vi "Panel Resized.vi"(6 "Sizing Refnums":T2, 8 "error in (no error)":errorcluster, 9 "Origin":cluster{"H":i16, "V":i16}, 10 "NewBnds":T1, 11 "Size Constraints":cluster{"min tab width":i32, "w/h":dbl}) -> (0 "error out":errorcluster)   [LabVIEW 2023]
uses:
  <vilib>/Utility/miscctls.llb/LVRectTypeDef.ctl
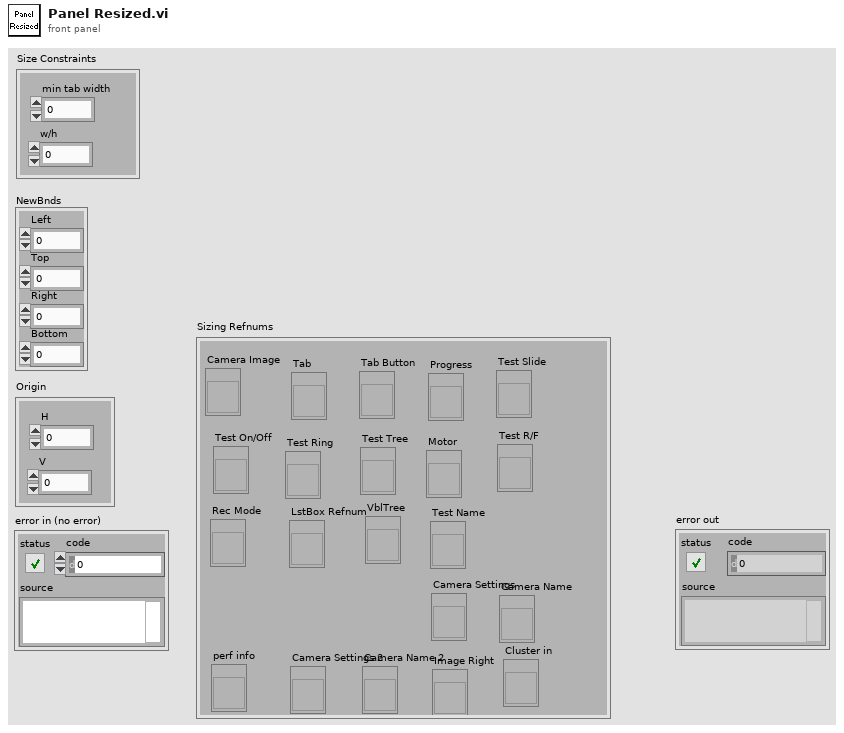
[diagram p1: front panel]
types:
  T1 = typedef "LVRectTypeDef.ctl" = cluster{"Left":i16, "Top":i16, "Right":i16, "Bottom":i16}
  T2 = cluster{"Camera Image":refnum<vi>, "Tab":refnum<vi>, "Tab Button":refnum<vi>, "Rec Mode":refnum<vi>, "Test Slide":refnum<vi>, "Test On/Off":refnum<vi>, "Test Ring":refnum<vi>, "Test R/F":refnum<vi>, "Test Name":refnum<vi>, "Motor":refnum<vi>, "Progress":refnum<vi>, "LstBox Refnum":refnum<vi>, "Test Tree":refnum<vi>, "VblTree":refnum<vi>, "Camera Settings":refnum<vi>, "Camera Name":refnum<vi>, "perf info":refnum<vi>, "Camera Settings 2":refnum<vi>, "Camera Name 2":refnum<vi>, "Image Right":refnum<vi>, "Cluster in":refnum<vi>}
  T3 = typedef "LVPositionTypeDef.ctl" = cluster{"Left":i32, "Top":i32}
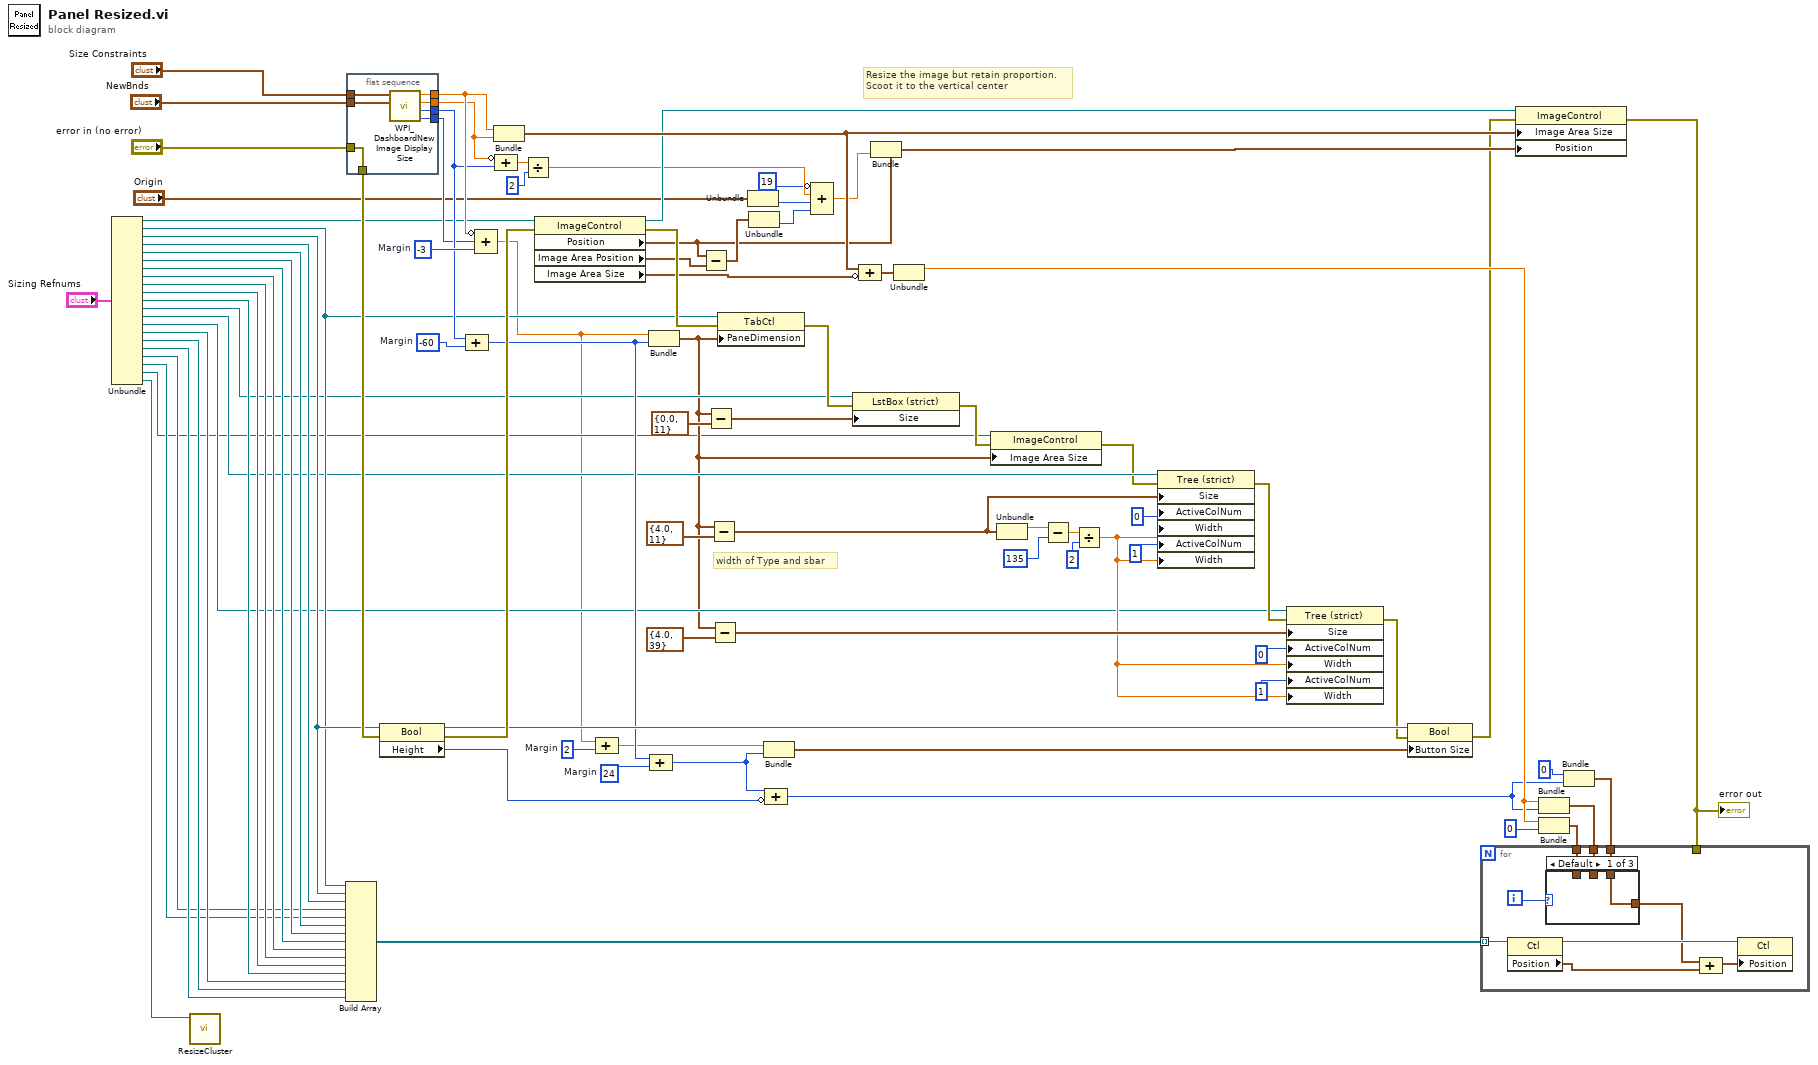
[diagram p0: block diagram]
diagram:
  w77 = 24  # Margin
  w75 = 2  # Margin
  w72 = -60  # Margin
  w81 = -3  # Margin
  # "width of Type and sbar"
  # "Resize the image but retain proportion.\nScoot it to the vertical center"
  n1 = Unbundle("Sizing Refnums") -> ("Camera Image"=w46:refnum<vi>, "Tab"=w47:refnum<vi>, "Tab Button"=w55:refnum<vi>, "Rec Mode"=w23:refnum<vi>, "Test Slide"=w22:refnum<vi>, "Test On/Off"=w21:refnum<vi>, "Test Ring"=w20:refnum<vi>, "Test R/F"=w19:refnum<vi>, "Test Name"=w18:refnum<vi>, "Motor"=w17:refnum<vi>, "Progress"=w16:refnum<vi>, "LstBox Refnum"=w15:refnum<vi>, "Test Tree"=w14:refnum<vi>, "VblTree"=w13:refnum<vi>, "Camera Settings"=w10:refnum<vi>, "Camera Name"=w9:refnum<vi>, "perf info"=w8:refnum<vi>, "Camera Settings 2"=w7:refnum<vi>, "Camera Name 2"=w6:refnum<vi>, "Image Right"=w3:refnum<vi>, "Cluster in"=w1:refnum<vi>)
  n2 = call "ResizeCluster.vi"("Cluster in"=w1) -> ()  [unwired: 11 in]
  n3 = Build Array(w47, w55, w23, w7, w6, w22, w21, w20, w19, w18, w17, w16, w10, w9, w8) -> (w90:refnum<vi>[])
  n4 = flat-sequence {
    tunnel: "NewBnds" -> [w97]
    tunnel: "Size Constraints" -> [w96]
    tunnel: [w95] -> w71
    tunnel: [w94] -> w78
    tunnel: [w93] -> w79
    tunnel: [w92] -> w80
    tunnel: [w91] -> w89
    tunnel: "error in (no error)" -> [w91]
    frame #0 {
      n5 = call <vilib>:"WPI_DashboardNew Image Display Size.vi"("NewBnds"=w97, "Size Constraints"=w96) -> ("Window Width"=w95:i16, "Window Height"=w93:i16, "Height"=w94:dbl, "Width"=w92:dbl)  [unwired: 6 in]
    }
  }
  n6 = property class="Bool"(reference=w55, error in=w89) -> (reference out=w84:refnum<vi>, error out=w88:errorcluster, "Height"=w83:u32)
  n7 = Compound Arithmetic op=unknown(w79, w72) -> (w76:i32)
  n8 = Compound Arithmetic op=ADD(invert w80, w71, w81) -> (w2:dbl)
  n9 = Bundle("Width"=w80, "Height"=w78) -> (w67:cluster{"Width":dbl, "Height":dbl})  [unwired: 1 in]
  n10 = Compound Arithmetic op=ADD(invert w78, w79) -> (w59:dbl)
  n11 = Divide(x=w59, y=2) -> (x/y=w61:dbl)
  n12 = property class="ImageControl"(reference=w46, error in=w88) -> (reference out=w64:refnum<vi>, error out=w87:errorcluster, "Position"=w63:T3, "Image Area Position"=w58:cluster{"Left":i32, "Top":i32}, "Image Area Size"=w69:cluster{"Width":u32, "Height":u32})
  n13 = Compound Arithmetic op=ADD(w2, w75) -> (w74:dbl)
  n14 = Bundle(w2, w76) -> (w12:cluster{dbl, i32})  [unwired: 1 in]
  n15 = Compound Arithmetic op=ADD(w76, w77) -> (w82:i32)
  n16 = Subtract(x=w63, y=w58) -> (x-y=w65:T3)
  n17 = Subtract(x=w12, y=cluster{dbl, i32} {0.0, 11}) -> (x-y=w44:cluster{dbl, i32})
  n18 = Subtract(x=w12, y=cluster{dbl, i32} {4.0, 11}) -> (x-y=w35:cluster{dbl, i32})
  n19 = Subtract(x=w12, y=cluster{dbl, i32} {4.0, 39}) -> (x-y=w40:cluster{dbl, i32})
  n20 = property class="TabCtl"(reference=w47, error in=w87, "PaneDimension"=w12) -> (error out=w45:errorcluster)  [unwired: 1 out]
  n21 = Unbundle("Origin") -> ("V"=w52:i16)  [unwired: 1 out]
  n22 = Unbundle(w65) -> ("Top"=w66:i32)  [unwired: 1 out]
  n23 = Bundle(w74, w82) -> (w73:cluster{dbl, i32})  [unwired: 1 in]
  n24 = Compound Arithmetic op=ADD(w82, invert w83) -> (w26:u32)
  n25 = Compound Arithmetic op=ADD(invert 19, w61, w52, w66) -> (w62:dbl)
  n26 = property class="LstBox (strict)"(reference=w15, error in=w45, "Size"=w44) -> (error out=w11:errorcluster)  [unwired: 1 out]
  n27 = Compound Arithmetic op=ADD(w67, invert w69) -> (w70:cluster{"Width":dbl, "Height":dbl})
  n28 = Bundle(cluster=w63, "Top"=w62) -> (w68:T3)  [unwired: 1 in]
  n29 = Unbundle(w70) -> ("Width"=w85:dbl)  [unwired: 1 out]
  n30 = property class="ImageControl"(reference=w3, error in=w11, "Image Area Size"=w12) -> (error out=w4:errorcluster)  [unwired: 1 out]
  n31 = Unbundle(w35) -> (w34:dbl)  [unwired: 1 out]
  n32 = Subtract(x=w34, y=135 ("Active Cell:Active Column Number")) -> (x-y=w30:dbl)
  n33 = Divide(x=w30, y=2 ("Active Cell:Active Column Number")) -> (x/y=w25:dbl)
  n34 = property class="Tree (strict)"(reference=w14, error in=w4, "Size"=w35, "ActiveColNum"=0 ("Active Cell:Active Column Number"), "Width"=w25, "ActiveColNum"=1 ("Active Cell:Active Column Number"), "Width"=w25) -> (error out=w39:errorcluster)  [unwired: 1 out]
  n35 = property class="Tree (strict)"(reference=w13, error in=w39, "Size"=w40, "ActiveColNum"=0 ("Active Cell:Active Column Number"), "Width"=w25, "ActiveColNum"=1 ("Active Cell:Active Column Number"), "Width"=w25) -> (error out=w38:errorcluster)  [unwired: 1 out]
  n36 = property class="Bool"(reference=w84, error in=w38, "Button Size"=w73) -> (error out=w5:errorcluster)  [unwired: 1 out]
  n37 = property class="ImageControl"(reference=w64, error in=w5, "Image Area Size"=w67, "Position"=w68) -> (error out=w51:errorcluster)  [unwired: 1 out]
  "error out" <- w51
  n38 = Bundle("Width"=w85, w26) -> (w57:cluster{"Width":dbl, u32})  [unwired: 1 in]
  n39 = Bundle("Width"=w85, 0) -> (w56:cluster{"Width":dbl, i32})  [unwired: 1 in]
  n40 = Bundle(0, w26) -> (w27:cluster{i32, u32})  [unwired: 1 in]
  n41 = for {
    tunnel: w90 -> [w106] mode=indexing
    tunnel: w57 -> [w100]
    tunnel: w56 -> [w101]
    tunnel: w51 -> [_]
    tunnel: w27 -> [w99]
    i -> [w102]
    n42 = property class="Ctl"(reference=w106) -> (reference out=w105:refnum<vi>, "Position"=w104:T3)  [unwired: 1 in, 1 out]
    n43 = case shown="Default" w102 {
      tunnel: w101 -> [_ w108 _]
      tunnel: w100 -> [_ _ w109]
      tunnel: w99 -> [w107 _ _]
      tunnel: [w107 w108 w109] -> w98
      frame Default {
      }
      frame 0, 1 {
      }
      frame 2..4 {
      }
    }
    n44 = Compound Arithmetic op=ADD(w98, w104) -> (w103:cluster{dbl, u32})
    n45 = property class="Ctl"(reference=w105, "Position"=w103) -> ()  [unwired: 1 in, 2 out]
  }
